vi "Show Spectrum Level.vi"(0 "Display State In":T1, 5 "Allow":bool, 9 "Container State":T2, 11 "error in (no error)":errorcluster) -> (4 "Display State Out":T1, 15 "error out":errorcluster)   [LabVIEW 2015, in "Level.xctl"]
uses:
  Level.xctl
  <vilib>/_xctls/Container State.ctl
  State.vi
  <vilib>/_xctls/XControlSupport.lvlib
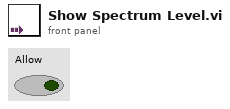
[diagram p1: front panel]
types:
  T1 = typedef "Level.xctl/State.vi" = cluster{"action":string, "excluded":enum16{"dB Atten", "dB Vrms", "dB SPL"}[]}
  T2 = typedef "XControlSupport.lvlib/Container State.ctl" = cluster{"Indicator?":bool, "Run Mode?":bool, " Refnum":refnum<vi>}
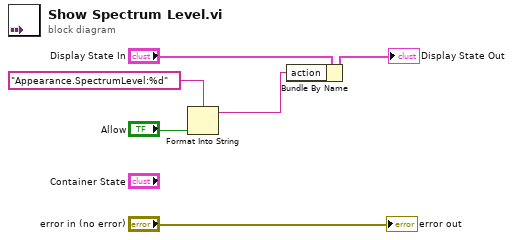
[diagram p0: block diagram]
diagram:
  n1 = Format Into String(format string="Appearance.SpectrumLevel:%d", "Allow") -> (resulting string=w1:string)  [unwired: 2 in, 1 out]
  n2 = Bundle By Name(cluster="Display State In", "action"=w1) -> (→"Display State Out":T1)
  "error out" <- "error in (no error)"
